vi "FIFORequests.vi"(1 "New One":T1, 2 "data out":string, 3 "Requests In":T2(array[cluster])) -> (0 "Requests Out":T2(array[cluster]))   [LabVIEW 2013]
uses:
  _ROSDefinition.vi
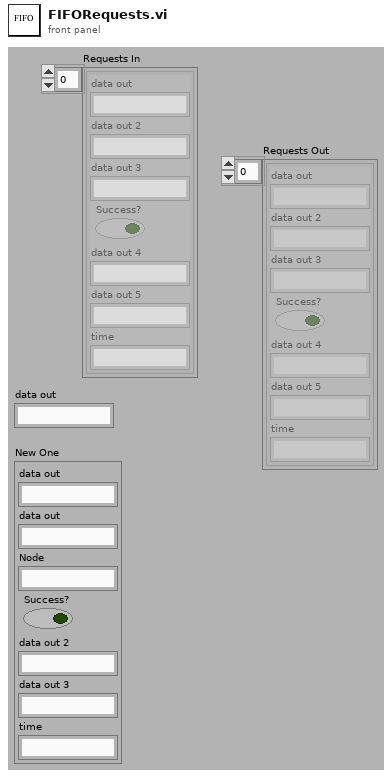
[diagram p1: front panel]
types:
  T1 = cluster{"data out":string, "data out":string, "Node":string, "Success?":bool, "data out 2":string, "data out 3":string, "time":string}
  T2 = cluster{"data out":string, "data out 2":string, "data out 3":string, "Success?":bool, "data out 4":string, "data out 5":string, "time":string}[]
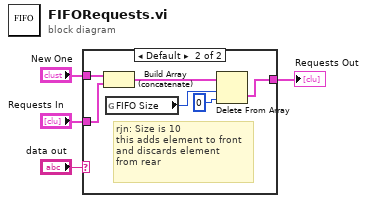
[diagram p0: block diagram]
diagram:
  n1 = case shown="Default" "data out" {
    tunnel: "New One" -> [_ w10]
    tunnel: "Requests In" -> [w5 w7]
    tunnel: [w5 w6] -> w1
    frame "" {
    }
    frame Default {
      # "rjn: Size is 10\nthis adds element to front\nand discards element\nfrom rear"
      n2 = Build Array (concatenate)(w10, w7) -> (w11:T2)
      n3 = global read "_ROSDefinition.vi" "FIFO Size"() -> (w8:i32)
      n4 = Delete From Array(array=w11, length=w8, index=0) -> (deleted portion=w6:T2)  [unwired: 1 out]
    }
  }
  "Requests Out" <- w1
